vi "set_field_current_with_backsweep.vi"(2 "Yokogawa Connection":T1={"Type"=1, "VISA"="TCPIP0::192.168.0.8::inst0::INSTR", "GPIB"="25"} {"Type" items=["VISA", "GPIB"]}, 3 "error in":errorcluster, 5 "I mA":dbl step=2e-05) -> (0 "error out":errorcluster)   [LabVIEW 2013]
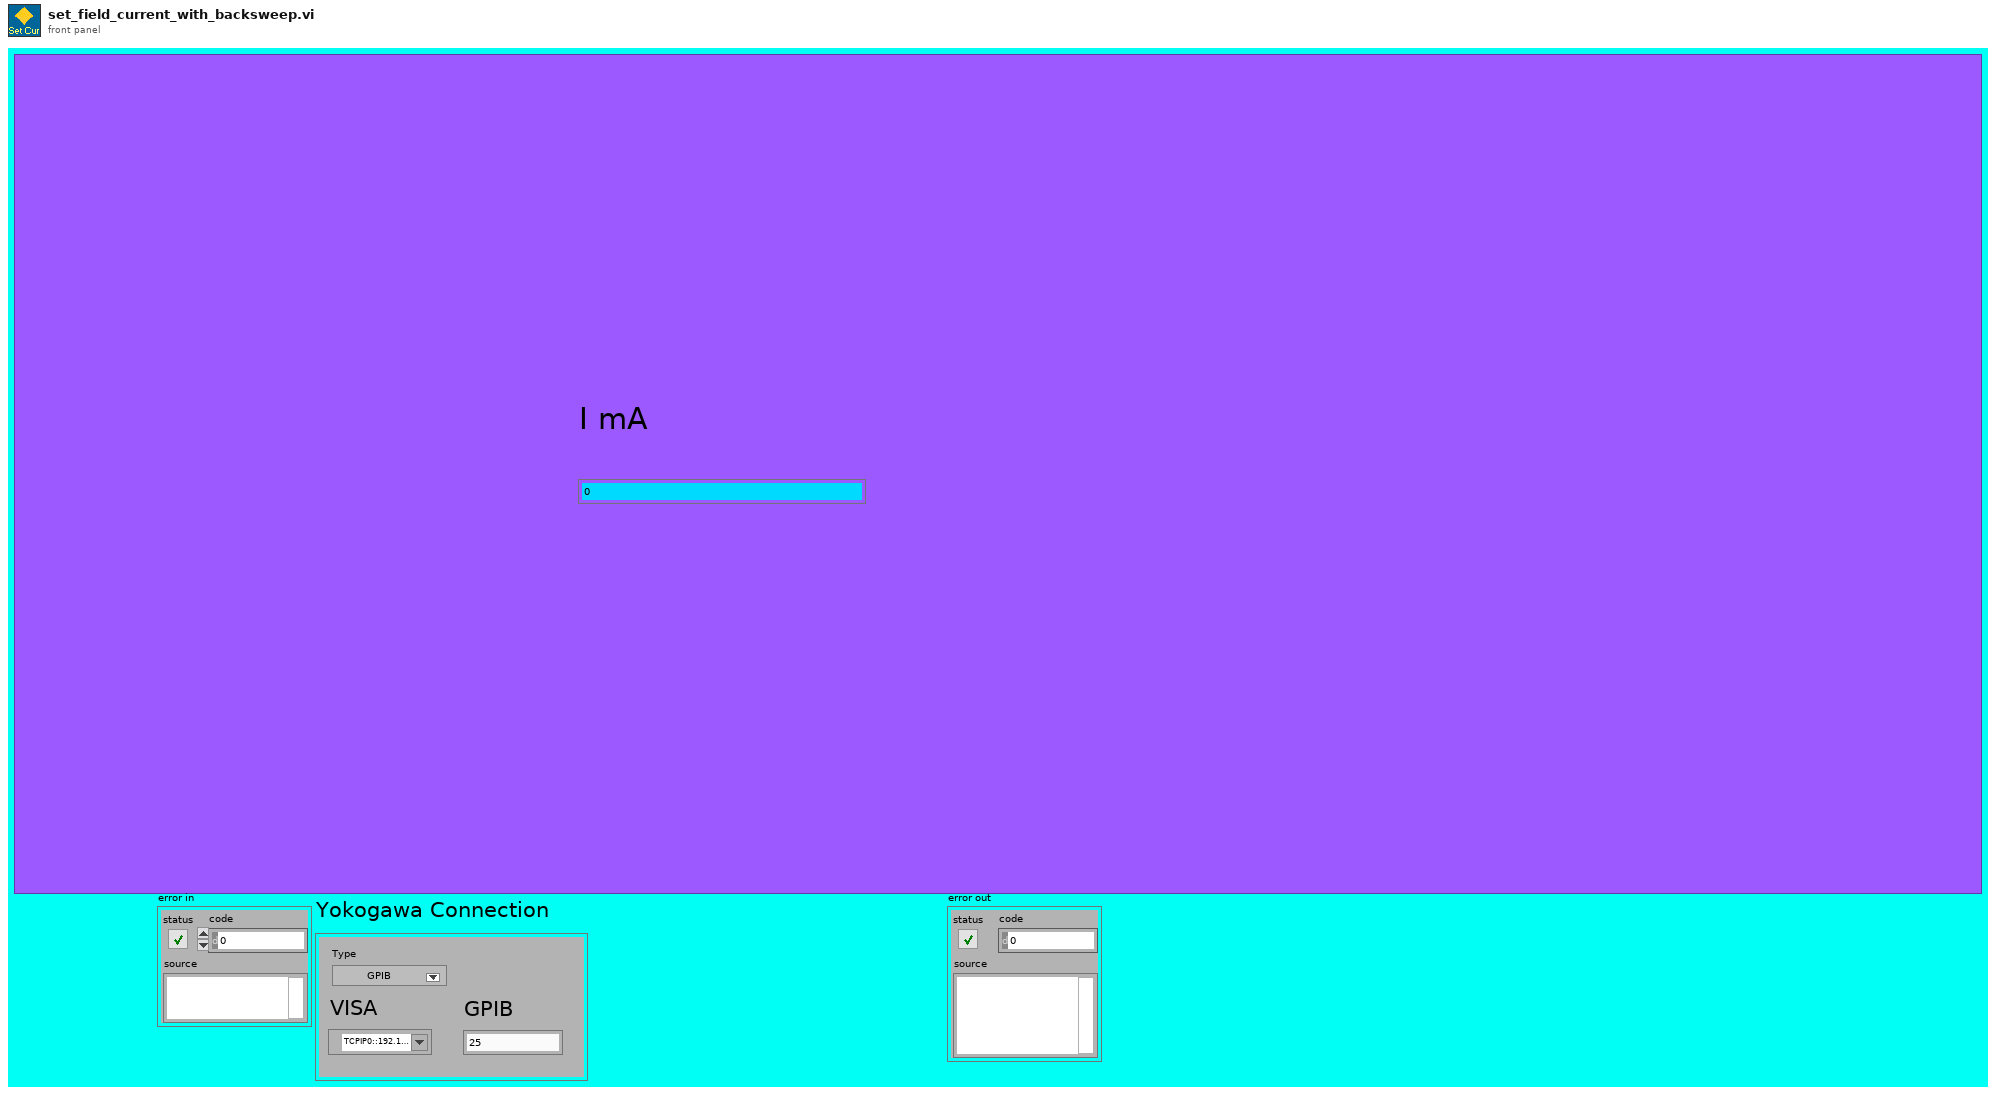
[diagram p1: front panel]
types:
  T1 = cluster{"Type":u16, "VISA":refnum<visa-resource-name>, "GPIB":string}
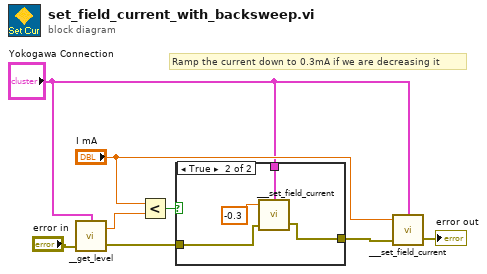
[diagram p0: block diagram]
diagram:
  # "Ramp the current down to 0.3mA if we are decreasing it"
  n1 = call "__get_level.vi"("Yokogawa Connection"="Yokogawa Connection", "error in"="error in") -> ("error out"=w6:errorcluster, "Current (mA)"=w8:dbl)  [unwired: 2 in]
  n2 = Less?(x="I mA", y=w8) -> (x < y?=w7:bool)
  n3 = case shown="True" w7 {
    tunnel: w6 -> [w9 w12]
    tunnel: [w9 w11] -> w4
    tunnel: "Yokogawa Connection" -> [_ w10]
    frame False {
    }
    frame True {
      n4 = call "___set_field_current.vi"("Yokogawa Connection"=w10, "error in"=w12, "I mA"=-0.3) -> ("error out"=w11:errorcluster)  [unwired: 1 in, 1 out]
    }
  }
  n5 = call "___set_field_current.vi"("Yokogawa Connection"="Yokogawa Connection", "error in"=w4, "I mA"="I mA") -> ("error out"=→"error out":errorcluster)  [unwired: 1 in, 1 out]
